vi "StandardStateMachine 1.vi"   [LabVIEW 2014]
doc: "Use this template to build a standard state machine design pattern. Each state executes code and determines which state to transition to. Contrast this design pattern with the User Interface Event Handler pattern, in which code executes in response to user actions. Contrast this design pattern also with the Queued Message Handler pattern, in which each message handling code can queue zero or more new messages.\nNote: This template does not contain the most recent programming guidelines recommended by National Instruments. For a complete, project-based implementation of the Standard State Machine pattern, use the Create Project dialog box instead of this template."
uses:
  TrajectoryGenerator.ctl
types:
  T1 = typedef "TrajectoryGenerator.ctl" = enum16{"Initialize", "Acceleration", "Correction A", "Constant Speed", "Deceleration", "Error", "Stop"}
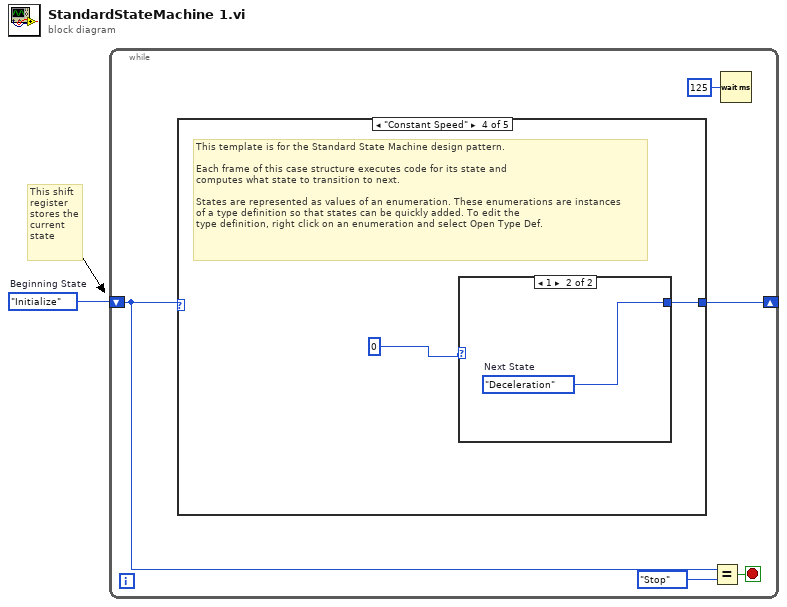
[diagram p0: block diagram]
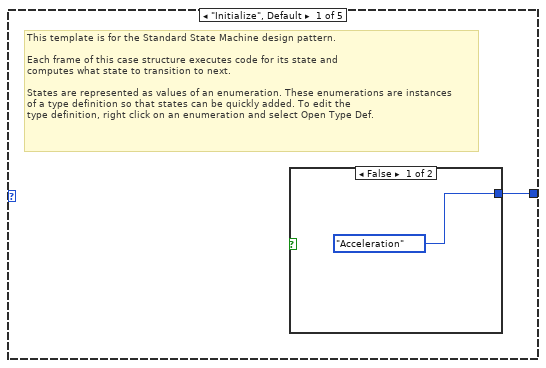
[diagram p2: hidden frame]
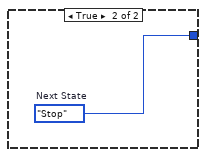
[diagram p3: hidden frame]
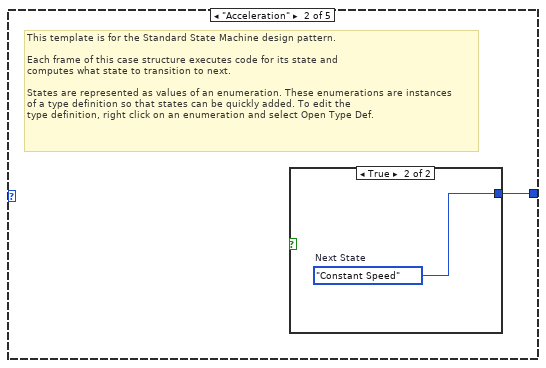
[diagram p4: hidden frame]
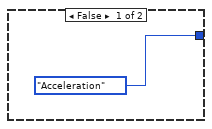
[diagram p5: hidden frame]
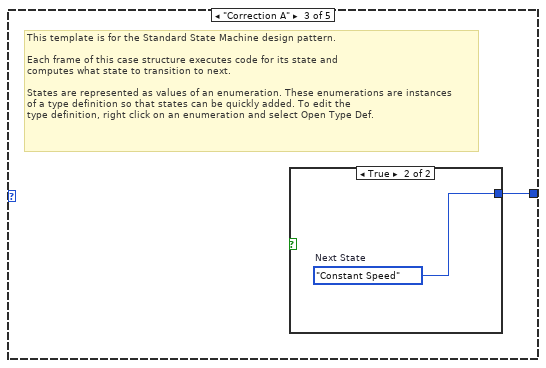
[diagram p6: hidden frame]
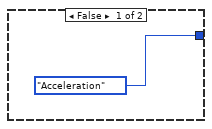
[diagram p7: hidden frame]
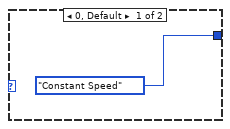
[diagram p8: hidden frame]
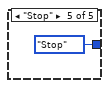
[diagram p9: hidden frame]
diagram:
  w1 = TrajectoryGenerator."Initialize"  # Beginning State
  # "This shift\nregister\nstores the\ncurrent\nstate"
  n1 = while {
    shift-right: [w3] -> _
    shift-left: w1 -> [w4]
    stop <- w6 stop-if-true
    n2 = case shown="\"Constant Speed\"" w4 {
      tunnel: [w7 w10 w13 w17 TrajectoryGenerator."Stop" ("Next State")] -> w3
      frame "Initialize", Default {
        # "This template is for the Standard State Machine design pattern.\n\nEach frame of this case structure executes code for its state and\ncomputes what state to transition to next.\n\nStates are represented as values of an enumeration. These enumerations are instances\nof a type definition so that states can be quickly added. To edit the \ntype definition, right click on an enumeration and select Open Type Def."
        n3 = case shown="False" {
          selector: _ -> [_ _]
          tunnel: [TrajectoryGenerator."Acceleration" ("Next State") w9] -> w7
          frame False {
          }
          frame True {
            w9 = TrajectoryGenerator."Stop"  # Next State
          }
        }
      }
      frame "Acceleration" {
        # "This template is for the Standard State Machine design pattern.\n\nEach frame of this case structure executes code for its state and\ncomputes what state to transition to next.\n\nStates are represented as values of an enumeration. These enumerations are instances\nof a type definition so that states can be quickly added. To edit the \ntype definition, right click on an enumeration and select Open Type Def."
        n4 = case shown="True" {
          selector: _ -> [_ _]
          tunnel: [TrajectoryGenerator."Acceleration" ("Next State") w12] -> w10
          frame False {
          }
          frame True {
            w12 = TrajectoryGenerator."Constant Speed"  # Next State
          }
        }
      }
      frame "Correction A" {
        # "This template is for the Standard State Machine design pattern.\n\nEach frame of this case structure executes code for its state and\ncomputes what state to transition to next.\n\nStates are represented as values of an enumeration. These enumerations are instances\nof a type definition so that states can be quickly added. To edit the \ntype definition, right click on an enumeration and select Open Type Def."
        n5 = case shown="True" {
          selector: _ -> [_ _]
          tunnel: [TrajectoryGenerator."Acceleration" ("Next State") w15] -> w13
          frame False {
          }
          frame True {
            w15 = TrajectoryGenerator."Constant Speed"  # Next State
          }
        }
      }
      frame "Constant Speed" {
        # "This template is for the Standard State Machine design pattern.\n\nEach frame of this case structure executes code for its state and\ncomputes what state to transition to next.\n\nStates are represented as values of an enumeration. These enumerations are instances\nof a type definition so that states can be quickly added. To edit the \ntype definition, right click on an enumeration and select Open Type Def."
        n6 = case shown="1" 0 {
          tunnel: [TrajectoryGenerator."Constant Speed" ("Next State") w19] -> w17
          frame 0, Default {
          }
          frame 1 {
            w19 = TrajectoryGenerator."Deceleration"  # Next State
          }
        }
      }
      frame "Stop" {
      }
    }
    n7 = Equal?(x=w4, y=TrajectoryGenerator."Stop" ("States")) -> (x = y?=w6:bool)
    n8 = Wait (ms)(milliseconds to wait=u32 125) -> ()  [unwired: 1 out]
  }
